vi "DCServoControl.vi"() -> ()   [LabVIEW 2019]
doc: "high-level user control for dc servo motor"
uses:
  D:/Victor Sun/optical trap control/Kinesis/Thorlabs.MotionControl.Controls.dll
  Kinesis/Thorlabs.MotionControl.Controls.dll
  D:/Victor Sun/optical trap control/Kinesis/ThorLabs.MotionControl.KCube.DCServoCLI.dll
  Kinesis/ThorLabs.MotionControl.KCube.DCServoCLI.dll
panel:
  in  "Folder path save":path
  in  "filename save":string="D:\\Victor Sun\\optical trap control\\output_test\\testposition"
  in  "stop data write loop":bool
  in  "start/stop write":bool
  in  "init file":bool
  out "current state":string
  out "Velocity":dbl
  out "OffsetDistance":dbl
  out "LimitSwitch":i32(ring) items=["Ignore"=0, "ClockwiseHard"=1, "CounterClockwiseHard"=4]
  out "Direction":i32(ring)=1 items=["Clockwise"=1, "CounterClockwise"=2]
  out "GotoAcceleration":dbl
  out "GotoMaxVelocity":dbl
  out "JogAcceleration":dbl
  out "JogMaxVelocity":dbl
  out "JogMode (this can not be controlled)":i16(ring)=1 items=["ContinuousHeld"=1, "SingleStep"=2, "ContinuousUnheld"=3]
  out "StopMode":i16(ring)=1 items=["Immediate"=1, "Profiled"=2]
  out "get absolute position":dbl
  out "backward step size":dbl
  out "forward step size":dbl
  out "backward position response limit":string
  out "Position Bar":dbl(slide) scale=0.0..25.0
  out "forward position response limit":string
  out "absolute position response limit":string
  in  "stop motors":bool
  in  "Go to position?":bool
  in  "Backward Button":bool
  in  "Forward Button":bool
  in  "absolute position":dbl
  in  "stepSize":dbl=0.1
  out "Position":dbl format="%_6g"
  in  "Stop Control Loop":bool
  in  "SerialNumber":string="27251750"
  in  "KCubeDCServoControl":refnum<k24>(container)
  # "Low-level parameters (not sure if to include controls for them)"
  # "Jog paras"
  # "Goto paras"
  # "Data Acquisition Settings"
  # "Absolute Position Control"
  # "Relative Position Control"
  # "Homing paras"
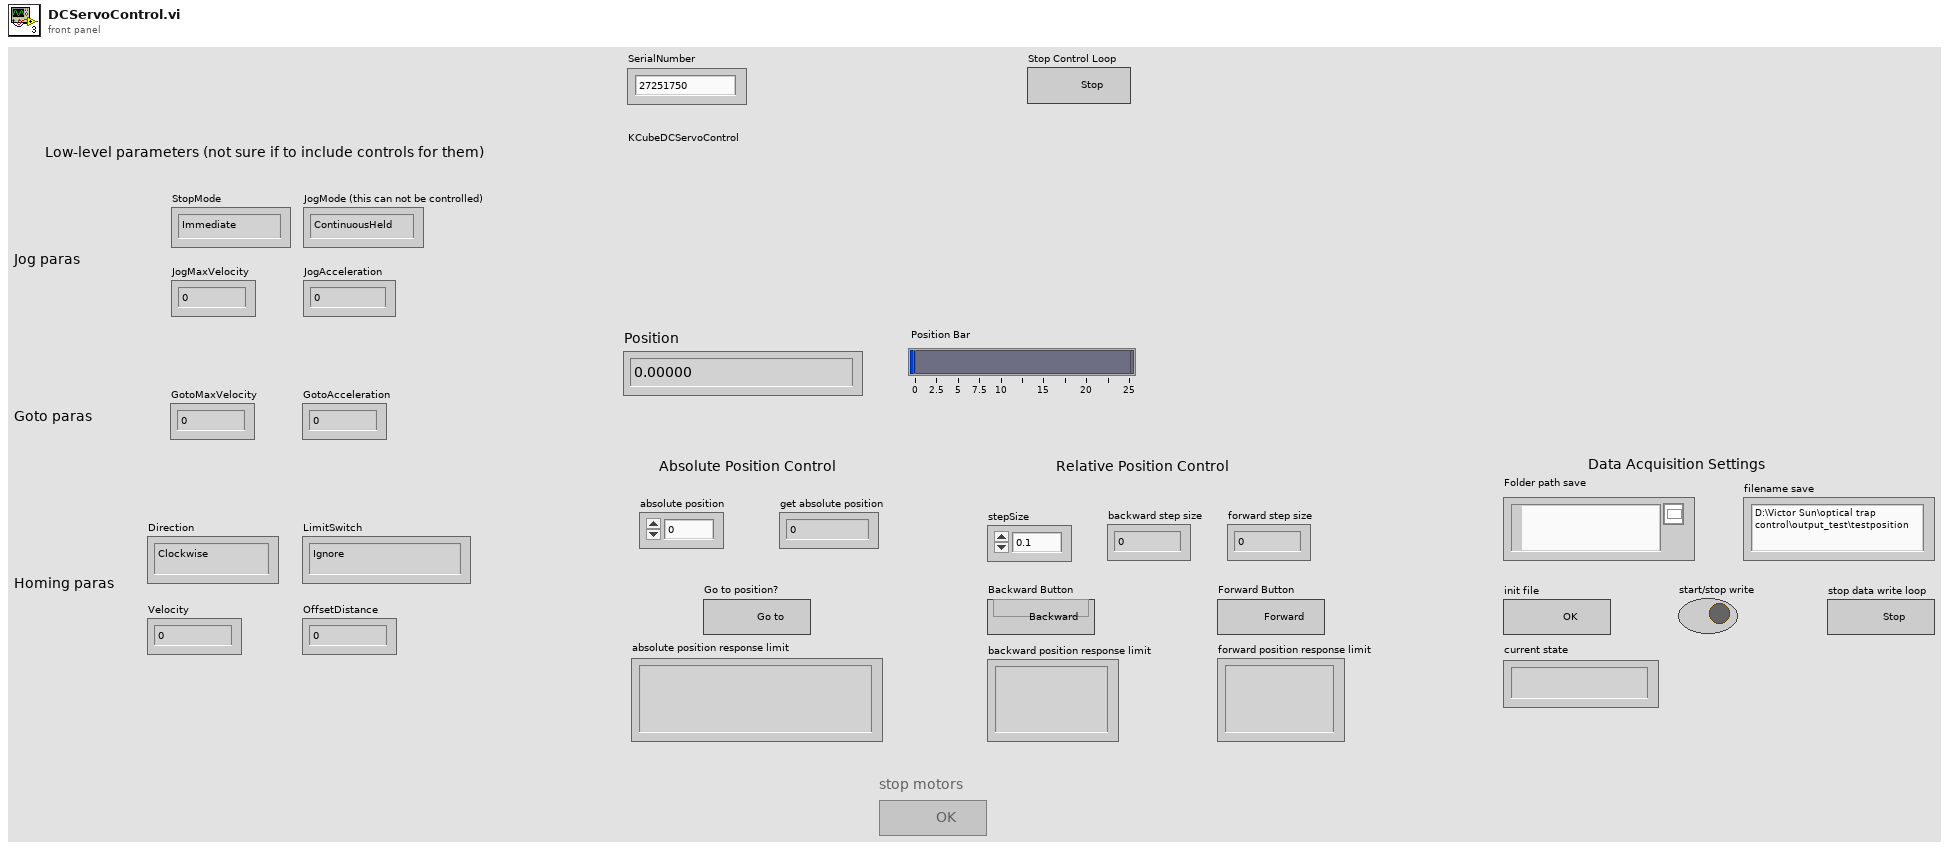
[diagram p1: front panel]
types:
  T1 = enum16{"waiting for init", "init", "waiting for write", "write", "stop"}
  T2 = enum8{"Enabled", "Disabled", "Disabled and Grayed Out"}
  T3 = cluster{"Velocity":dbl, "Direction":i32, "OffsetDistance":dbl, "LimitSwitch":i32}
  T4 = cluster{"StopMode":i16, "Acceleration":dbl, "MaxVelocity":dbl, "JogMode":i16}
  T5 = enum16{"waiting for init", "init", "waiting for write", "write", "stop", ""}
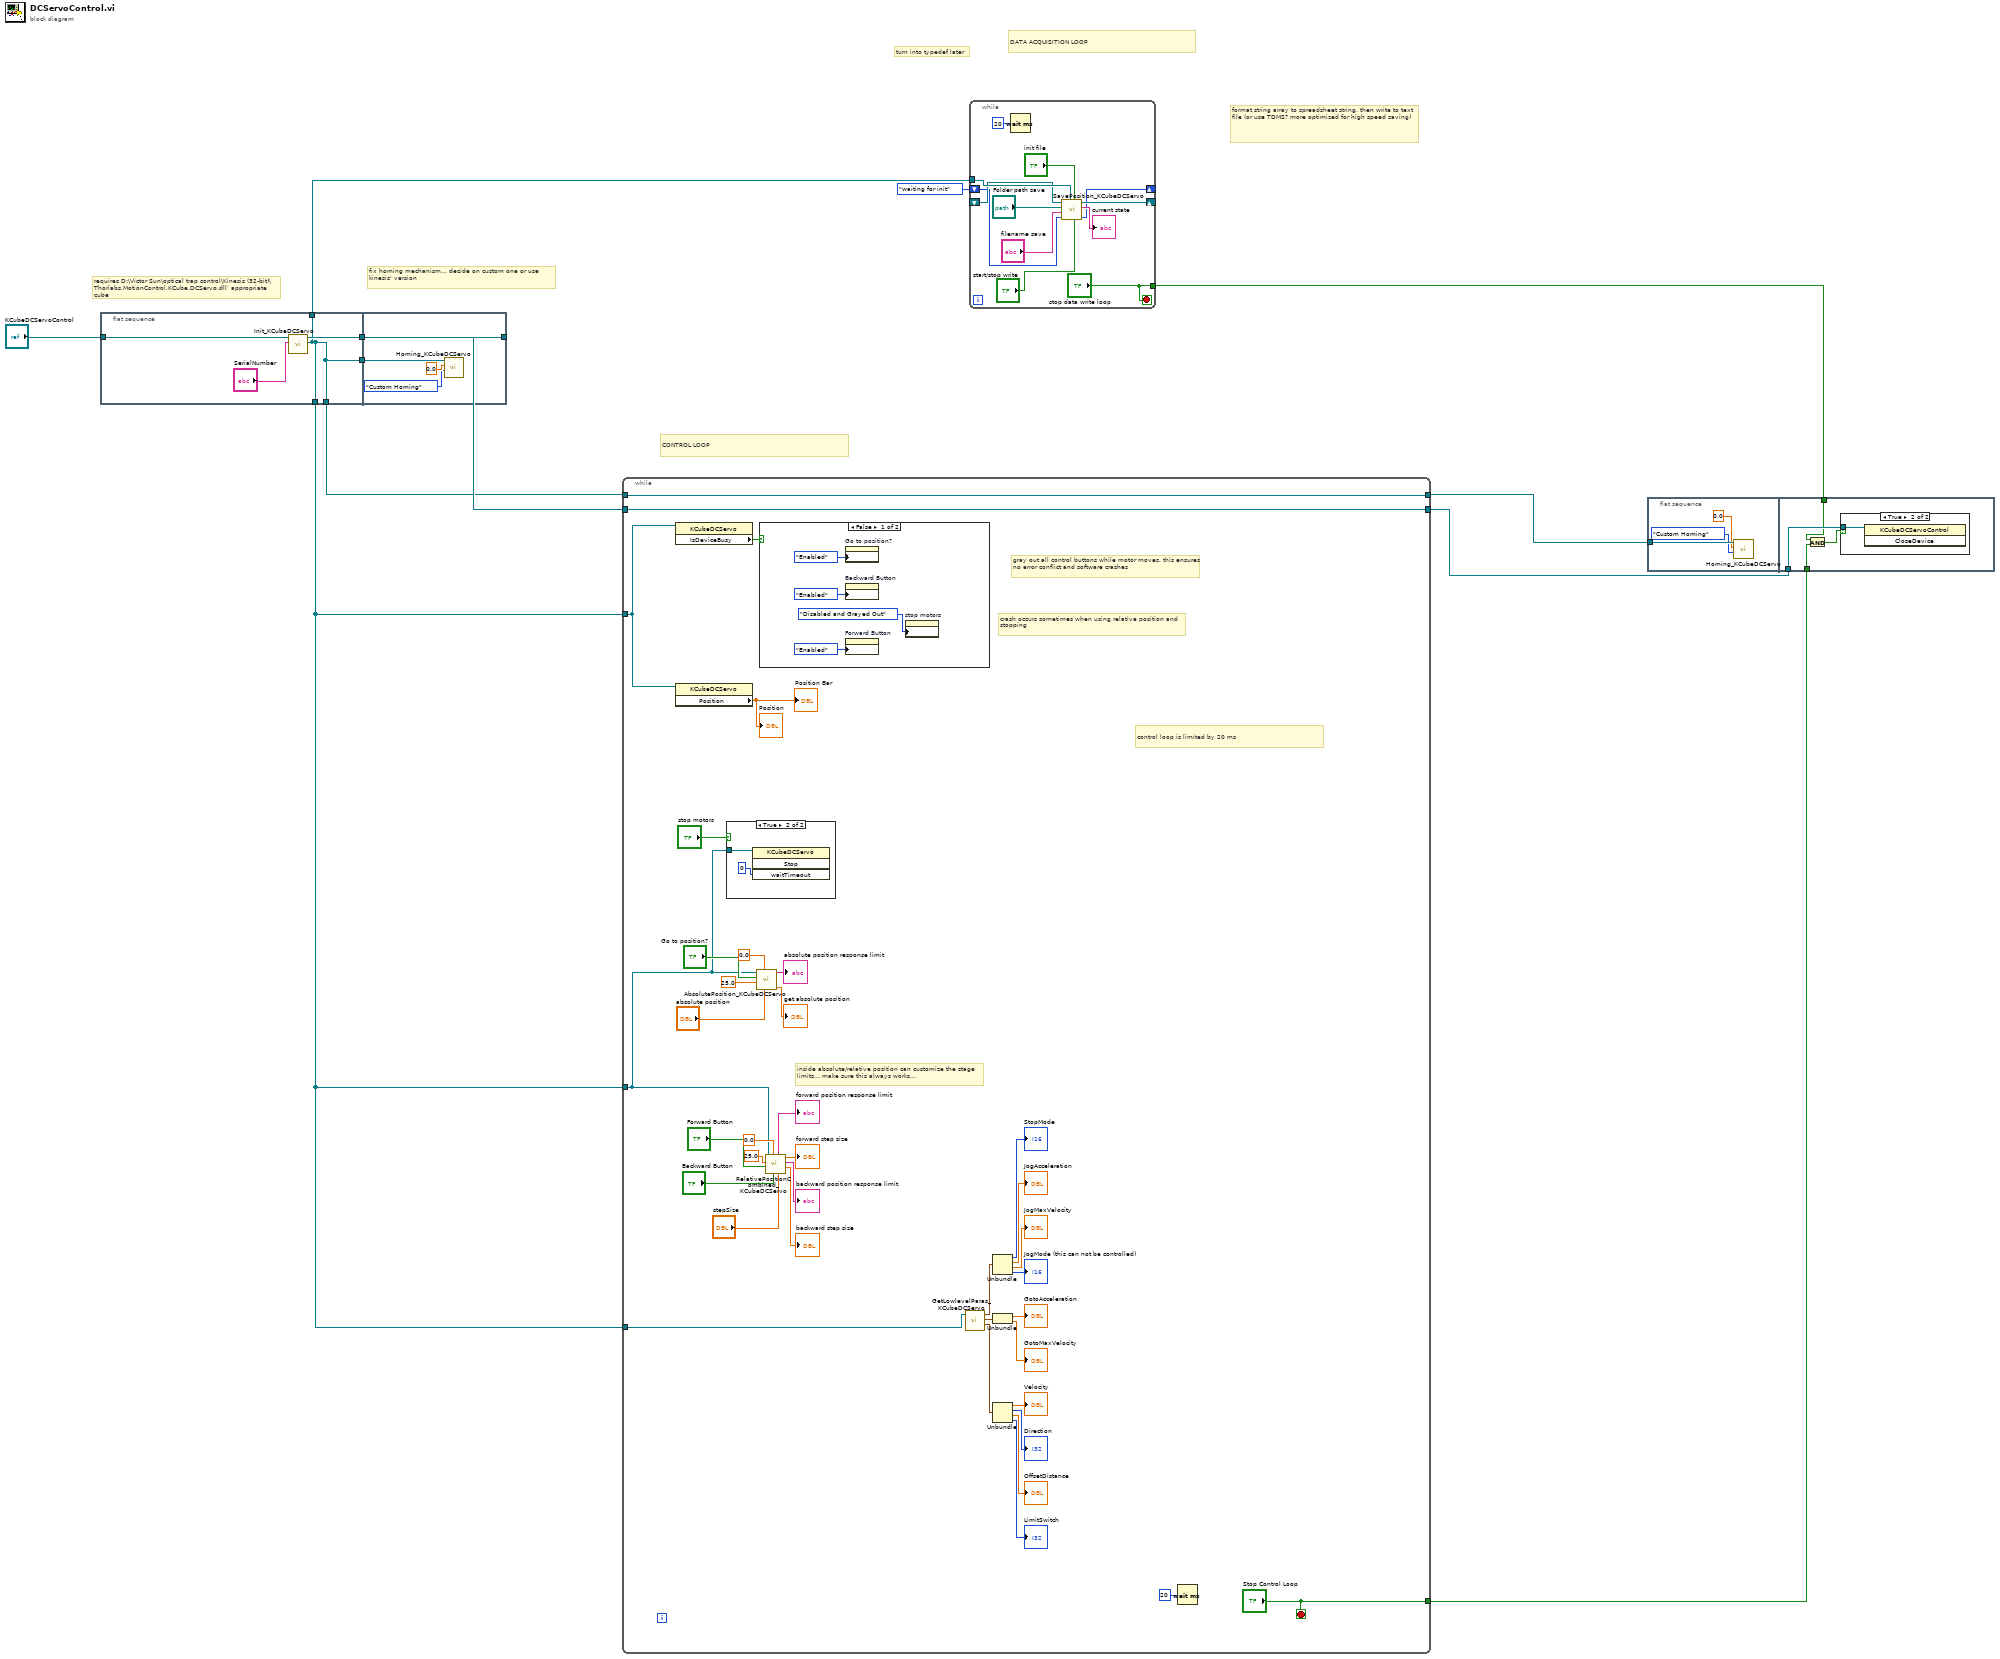
[diagram p0: block diagram]
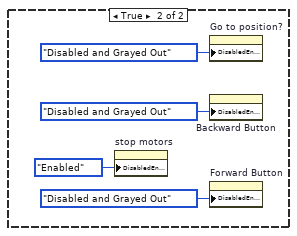
[diagram p3: hidden frame]
diagram:
  # "turn into typedef later"
  # "format string array to spreadsheet string, then write to text file (or use TDMS? more optimized for high speed saving)"
  # "DATA ACQUISITION LOOP"
  # "CONTROL LOOP"
  # "fix homing mechanism... decide on custom one or use kinesis' version"
  # "requires D:\\Victor Sun\\optical trap control\\Kinesis (32-bit)\\Thorlabs.MotionControl.KCube.DCServo.dll’ appropriate cube"
  n1 = flat-sequence {
    tunnel: "KCubeDCServoControl" -> [w16]
    tunnel: [w13] -> w10
    tunnel: [w14] -> w9
    tunnel: [w13] -> w8
    tunnel: [w13] -> w7
    tunnel: [w13] -> w3
    tunnel: [w20] -> w11
    tunnel: w9 -> [w20]
    tunnel: w8 -> [w18]
    frame #0 {
      n2 = call "Init_KCubeDCServo.vi"("SerialNumber"="SerialNumber", ".NET Refnum in"=w16) -> ("Device"=w13:refnum<k24>, ".NET Refnum out"=w14:refnum<k24>)  [unwired: 7 in, 1 out]
    }
    frame #1 {
      n3 = call "Homing_KCubeDCServo.vi"("Homing type"=enum16{"Custom Homing", "Kinesis Homing"}."Custom Homing", "set absolute position"=0.0 ("position"), ".NET Refnum in"=w18) -> ()  [unwired: 7 in, 2 out]
    }
  }
  n4 = while {
    tunnel: w11 -> [w58]
    tunnel: [w58] -> w5
    tunnel: w10 -> [w22]
    tunnel: w10 -> [w54]
    tunnel: w10 -> [w36]
    tunnel: w7 -> [w37]
    tunnel: [w37] -> w6
    tunnel: ["Stop Control Loop"] -> w1
    stop <- "Stop Control Loop" stop-if-true
    # "control loop is limited by 20 ms"
    # "crash occurs sometimes when using relative position and stopping"
    # "gray out all control buttons while motor moves. this ensures no error conflict and software crashes"
    # "inside absolute/relative position can customize the stage limits... make sure this always works..."
    n5 = property class="KCubeDCServo"(reference=w54) -> ("IsDeviceBusy"=w53:bool)  [unwired: 1 in, 2 out]
    n6 = property class="KCubeDCServo"(reference=w54) -> ("Position"=→"Position" →"Position Bar":dbl)  [unwired: 1 in, 2 out]
    n7 = case shown="True" "stop motors" {
      tunnel: w22 -> [_ w67]
      frame False {
      }
      frame True {
        n8 = invoke class="KCubeDCServo" method="Stop"(reference=w67, "waitTimeout"=0) -> ()  [unwired: 2 in, 4 out]
      }
    }
    n9 = call "AbsolutePosition_KCubeDCServo.vi"("set absolute position"="absolute position", "lower limit"=0.0, "upper limit"=25.0, "go to button"="Go to position?", ".NET Refnum in"=w22) -> ("get absolute position"=→"get absolute position":dbl, "absolute position response limit"=→"absolute position response limit":string)  [unwired: 5 in]
    n10 = case shown="False" w53 {
      frame False {
        n11 = property on="Go to position?" class="Bool"("DisabledEnum"=T2."Enabled" ("Disabled")) -> ()  [unwired: 2 in, 2 out]
        n12 = property on="Backward Button" class="Bool"("DisabledEnum"=T2."Enabled" ("Disabled")) -> ()  [unwired: 2 in, 2 out]
        n13 = property on="Forward Button" class="Bool"("DisabledEnum"=T2."Enabled" ("Disabled")) -> ()  [unwired: 2 in, 2 out]
        n14 = property on="stop motors" class="Bool"("DisabledEnum"=T2."Disabled and Grayed Out" ("Disabled")) -> ()  [unwired: 2 in, 2 out]
      }
      frame True {
        n15 = property on="stop motors" class="Bool"("DisabledEnum"=T2."Enabled" ("Disabled")) -> ()  [unwired: 2 in, 2 out]
        n16 = property on="Go to position?" class="Bool"("DisabledEnum"=T2."Disabled and Grayed Out" ("Disabled")) -> ()  [unwired: 2 in, 2 out]
        n17 = property on="Backward Button" class="Bool"("DisabledEnum"=T2."Disabled and Grayed Out" ("Disabled")) -> ()  [unwired: 2 in, 2 out]
        n18 = property on="Forward Button" class="Bool"("DisabledEnum"=T2."Disabled and Grayed Out" ("Disabled")) -> ()  [unwired: 2 in, 2 out]
      }
    }
    n19 = call "RelativePositionCombined_KCubeDCServo.vi"("stepSize"="stepSize", "Backward Button"="Backward Button", "lower limit"=0.0, "Forward Button"="Forward Button", "upper limit"=25.0, ".NET Refnum in"=w22) -> ("backward step size"=→"backward step size":dbl, "backward position response limit"=→"backward position response limit":string, "forward step size"=→"forward step size":dbl, "forward position response limit"=→"forward position response limit":string)  [unwired: 2 in]
    n20 = call "GetLowlevelParas_KCubeDCServo.vi"(".NET Refnum in"=w36) -> ("Cluster 2"=w30:T3, "Cluster"=w25:cluster{"Acceleration":dbl, "MaxVelocity":dbl}, "Cluster 3"=w35:T4)  [unwired: 8 in]
    n21 = Unbundle(w35) -> ("StopMode"=→"StopMode":i16, "Acceleration"=→"JogAcceleration":dbl, "MaxVelocity"=→"JogMaxVelocity":dbl, "JogMode"=→"JogMode (this can not be controlled)":i16)
    n22 = Unbundle(w25) -> ("Acceleration"=→"GotoAcceleration":dbl, "MaxVelocity"=→"GotoMaxVelocity":dbl)
    n23 = Unbundle(w30) -> ("Velocity"=→"Velocity":dbl, "Direction"=→"Direction":i32, "OffsetDistance"=→"OffsetDistance":dbl, "LimitSwitch"=→"LimitSwitch":i32)
    n24 = Wait (ms)(milliseconds to wait=u32 20) -> ()  [unwired: 1 out]
  }
  n25 = while {
    shift-right: [w69] -> _
    shift-left: T1."waiting for init" -> [w70]
    tunnel: w3 -> [w78]
    shift-right: [w77] -> _
    shift-left: _ -> [w76]
    tunnel: ["stop data write loop"] -> w2
    stop <- "stop data write loop" stop-if-true
    n26 = Wait (ms)(milliseconds to wait=u32 20) -> ()  [unwired: 1 out]
    n27 = call "SavePosition_KCubeDCServo.vi"("start/stop write"="start/stop write", "init file"="init file", "Device"=w78, "state in"=w70, "filename save"="filename save", "folder path save"="Folder path save", "Byte Stream File in"=w76) -> ("state out"=w69:T5, "current state"=→"current state":string, "Byte Stream File out"=w77:refnum<file>)  [unwired: 2 in]
  }
  n28 = flat-sequence {
    tunnel: w6 -> [w83]
    tunnel: w5 -> [w87]
    tunnel: w2 -> [w85]
    tunnel: w1 -> [w84]
    frame #0 {
      n29 = call "Homing_KCubeDCServo.vi"("Homing type"=enum16{"Custom Homing", "Kinesis Homing"}."Custom Homing", "set absolute position"=0.0 ("position"), ".NET Refnum in"=w83) -> ()  [unwired: 7 in, 2 out]
    }
    frame #1 {
      n30 = And(x=w85, y=w84) -> (x .and. y?=w86:bool)
      n31 = case shown="True" w86 {
        tunnel: w87 -> [_ w88]
        frame False {
        }
        frame True {
          n32 = invoke class="KCubeDCServoControl" method="CloseDevice"(reference=w88) -> ()  [unwired: 2 in, 3 out]
        }
      }
    }
  }
